vi "LV SciSDK LIST START.vi"(0 "List name":string, 4 "Handle In":T2, 5 "error in (no error)":errorcluster) -> (18 "CP Handle Out":T1)   [LabVIEW 2021]
uses:
  SciSDK_Labview.lvlib
panel:
  out "error out":errorcluster
  in  "Threaded Buffer Size":u32=100000
  in  "High Performance":string(combo)="false"
  in  "Thread":string(combo)="false"
  in  "Timeout":i32=100
  in  "Acq Mode":string(combo)="blocking"
  in  "Acq Len":u32=1024
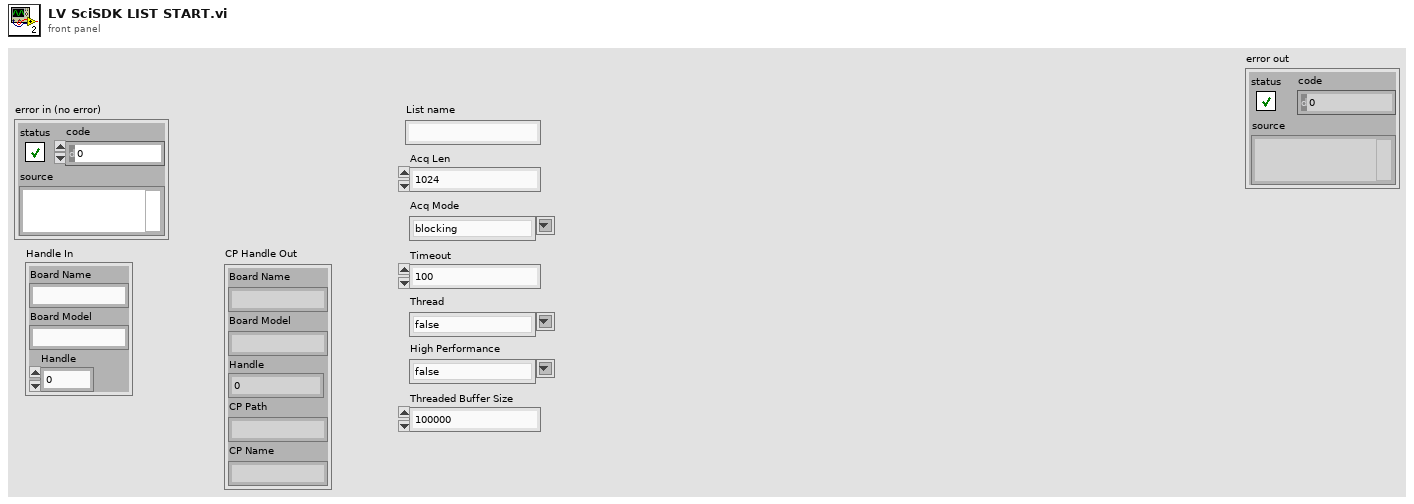
[diagram p1: front panel]
types:
  T1 = cluster{"Board Name":string, "Board Model":string, "Handle":u64, "CP Path":string, "CP Name":string}
  T2 = cluster{"Board Name":string, "Board Model":string, "Handle":u64}
  T3 = cluster{"Board Name":string, "Board Model":string, "Handle":u64, string, "List name":string}
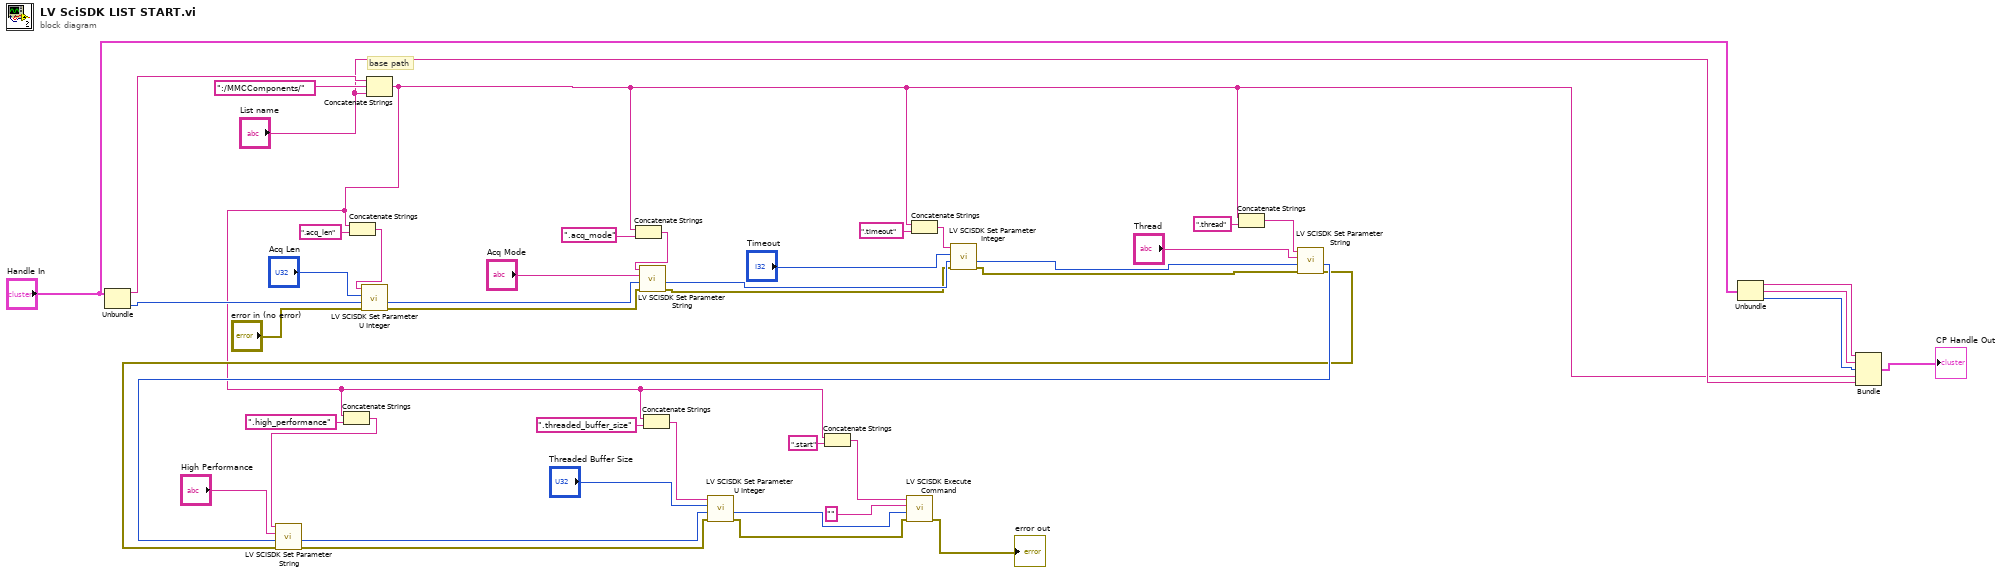
[diagram p0: block diagram]
diagram:
  # "base path"
  n1 = Unbundle("Handle In") -> ("Board Name"=w40:string, "Handle"=w27:u64)  [unwired: 1 out]
  n2 = Concatenate Strings(w40, ":/MMCComponents/" ("string"), "List name") -> (w1:string)
  n3 = Concatenate Strings(w1, ".high_performance" ("string")) -> (w14:string)
  n4 = Concatenate Strings(w1, ".acq_len" ("string")) -> (w29:string)
  n5 = call "LV SCISDK Set Parameter U Integer.vi"("error in (no error)"="error in (no error)", "handle"=w27, "value"="Acq Len", "Path"=w29) -> ("error out"=w24:errorcluster, "handle out"=w25:u64)  [unwired: 5 in, 1 out]
  n6 = Concatenate Strings(w1, ".acq_mode" ("string")) -> (w31:string)
  n7 = call "LV SCISDK Set Parameter String.vi"("error in (no error)"=w24, "handle"=w25, "value"="Acq Mode", "Path"=w31) -> ("error out"=w20:errorcluster, "handle out"=w21:u64)  [unwired: 5 in, 1 out]
  n8 = Concatenate Strings(w1, ".threaded_buffer_size" ("string")) -> (w11:string)
  n9 = Concatenate Strings(w1, ".start" ("string")) -> (w4:string)
  n10 = Concatenate Strings(w1, ".timeout" ("string")) -> (w23:string)
  n11 = call "LV SCISDK Set Parameter Integer.vi"("error in (no error)"=w20, "handle"=w21, "value"="Timeout", "Path"=w23) -> ("error out"=w16:errorcluster, "handle out"=w17:u64)  [unwired: 5 in, 1 out]
  n12 = Concatenate Strings(w1, ".thread" ("string")) -> (w18:string)
  n13 = call "LV SCISDK Set Parameter String.vi"("error in (no error)"=w16, "handle"=w17, "value"="Thread", "Path"=w18) -> ("error out"=w12:errorcluster, "handle out"=w13:u64)  [unwired: 5 in, 1 out]
  n14 = call "LV SCISDK Set Parameter String.vi"("error in (no error)"=w12, "handle"=w13, "value"="High Performance", "Path"=w14) -> ("error out"=w8:errorcluster, "handle out"=w9:u64)  [unwired: 5 in, 1 out]
  n15 = call "LV SCISDK Set Parameter U Integer.vi"("error in (no error)"=w8, "handle"=w9, "value"="Threaded Buffer Size", "Path"=w11) -> ("error out"=w7:errorcluster, "handle out"=w2:u64)  [unwired: 5 in, 1 out]
  n16 = call "LV SCISDK Execute Command.vi"("error in (no error)"=w7, "handle"=w2, "value"="", "Path"=w4) -> ("error out"=→"error out":errorcluster)  [unwired: 5 in, 2 out]
  n17 = Unbundle("Handle In") -> ("Board Name"=w43:string, "Board Model"=w42:string, "Handle"=w41:u64)
  n18 = Bundle("Board Name"=w43, "Board Model"=w42, "Handle"=w41, w1, "List name"="List name") -> (→"CP Handle Out":T3)  [unwired: 1 in]
